vi "Read Name Dependecy.vi"(8 "error in (no error)":errorcluster, 11 "Mapping Column in":refnum<class "Mapping Column.lvclass">) -> (0 "error out":errorcluster, 2 "Name Dependecy":i32, 3 "Mapping Column out":refnum<class "Mapping Column.lvclass">)   [LabVIEW 2013, in "Table Manager.lvlib" / "Mapping Column.lvclass"]
uses:
  Mapping Column.lvclass
  Mapping Column.lvclass/Mapping Column.ctl
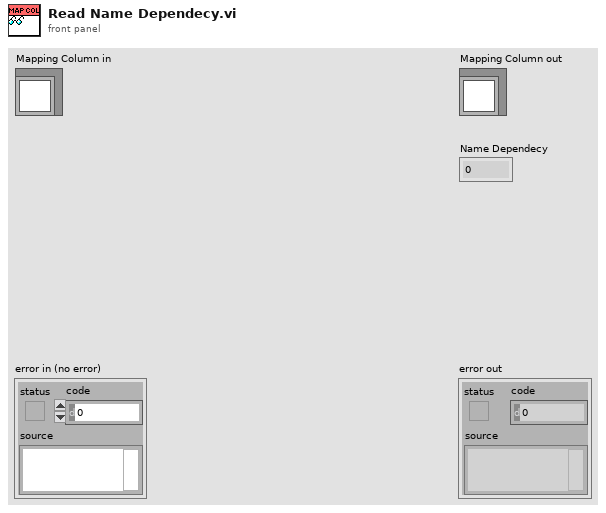
[diagram p1: front panel]
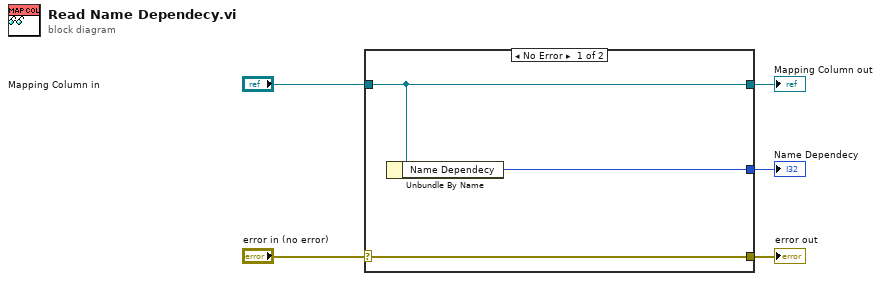
[diagram p0: block diagram]
diagram:
  n1 = case shown="No Error" "error in (no error)" {
    selector: "error in (no error)" -> [w8 w9]
    tunnel: [w8 w9] -> w4
    tunnel: [w7 w10] -> w2
    tunnel: "Mapping Column in" -> [w7 w10]
    tunnel: [w6 _] -> w1
    frame No Error {
      n2 = Unbundle By Name(w7) -> ("Name Dependecy"=w6:i32)
    }
    frame Error {
    }
  }
  "error out" <- w4
  "Mapping Column out" <- w2
  "Name Dependecy" <- w1
